vi "Tree Deep Copy Item.vi"(4 "Erase Target Tree":bool=TRUE, 6 "Parent Tag":string, 8 "error in":errorcluster, 9 "Target Tree Ref In":refnum<vi>, 10 "Target Item":string, 11 "Source Tree Ref In":refnum<vi>) -> (0 "error out":errorcluster, 1 "Target Tree Ref Out":refnum<vi>, 3 "Source Tree Ref Out":refnum<vi>)   [LabVIEW 2024]
uses:
  Tree Copy Single Item.vi
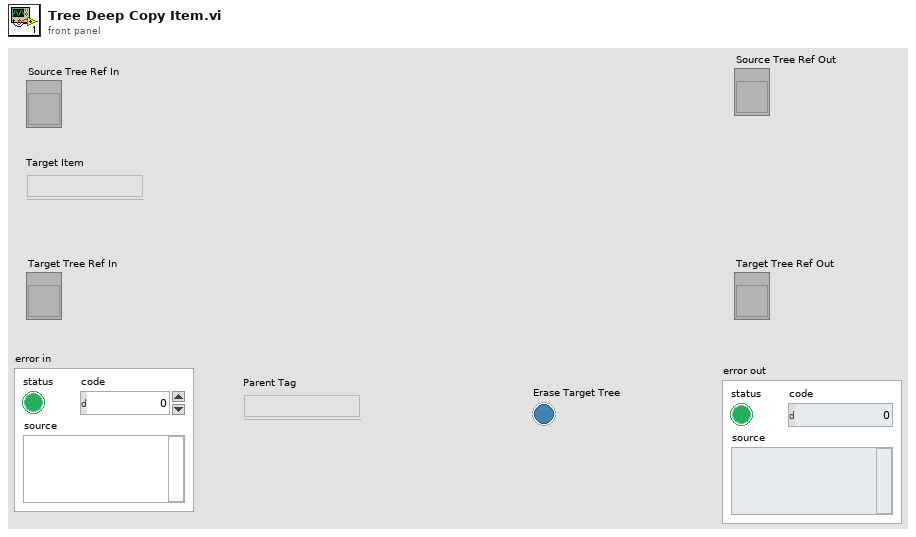
[diagram p1: front panel]
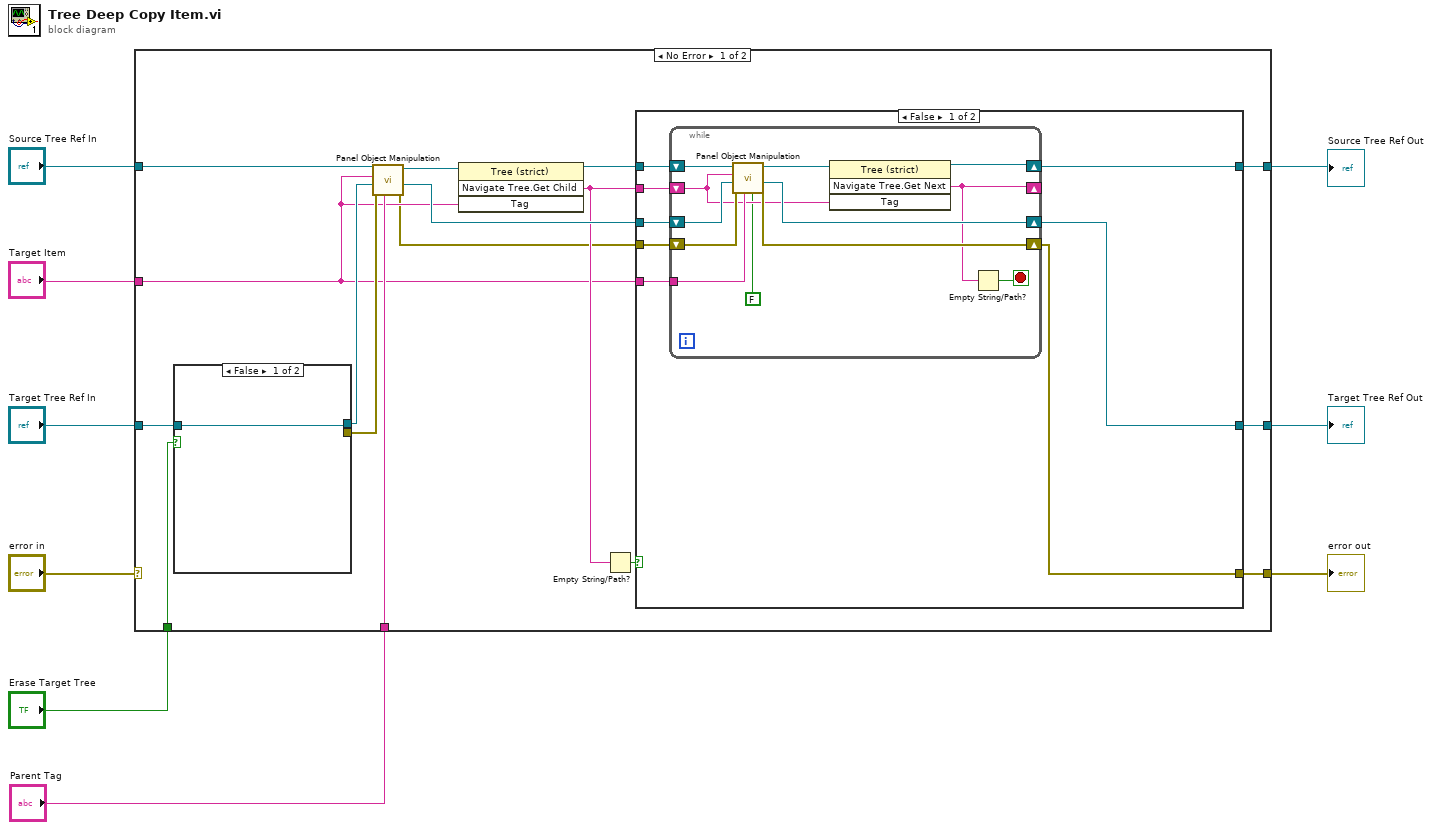
[diagram p0: block diagram]
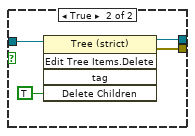
[diagram p3: hidden frame]
diagram:
  n1 = case shown="No Error" "error in" {
    selector: "error in" -> [_ w55]
    tunnel: [w10 w55] -> w8
    tunnel: "Target Tree Ref In" -> [w25 w53]
    tunnel: "Erase Target Tree" -> [w24 _]
    tunnel: "Target Item" -> [w12 _]
    tunnel: "Source Tree Ref In" -> [w23 w54]
    tunnel: "Parent Tag" -> [w20 _]
    tunnel: [w16 w54] -> w3
    tunnel: [w14 w53] -> w2
    frame No Error {
      n2 = case shown="False" w24 {
        tunnel: w25 -> [w48 w51]
        tunnel: [w48 w50] -> w22
        tunnel: [_ w49] -> w17
        frame False {
        }
        frame True {
          n3 = invoke class="Tree (strict)" method="Edit Tree Items.Delete"(reference=w51, "Delete Children"=TRUE ("Delete Children?")) -> (reference out=w50:refnum<vi>, error out=w49:errorcluster)  [unwired: 3 in, 3 out]
        }
      }
      n4 = call-poly "Panel Object Manipulation.vi"("Parent Tag"=w20, "error in"=w17, "Target Tree Ref In"=w22, "Target Item"=w12, "Source Tree Ref In"=w23) -> ("error out"=w11:errorcluster, "Target Tree Ref Out"=w15:refnum<vi>, "Source Tree Ref Out"=w21:refnum<vi>)  [unwired: 4 in]
      n5 = invoke class="Tree (strict)" method="Navigate Tree.Get Child"(reference=w21, "Tag"=w12) -> (reference out=w19:refnum<vi>, "Navigate Tree:Get Child"=w13:string)  [unwired: 2 in, 2 out]
      n6 = Empty String/Path?(string/path=w13) -> (empty?=w18:bool)
      n7 = case shown="False" w18 {
        tunnel: w19 -> [w33 w47]
        tunnel: [w29 w47] -> w16
        tunnel: w15 -> [w31 w46]
        tunnel: [w28 w46] -> w14
        tunnel: w13 -> [w32 _]
        tunnel: w12 -> [w30 _]
        tunnel: w11 -> [w27 _]
        tunnel: [w26 _] -> w10
        frame False {
          n8 = while {
            tunnel: w30 -> [w43]
            shift-right: [w38] -> w29
            shift-left: w33 -> [w45]
            shift-right: [w42] -> w28
            shift-left: w31 -> [w44]
            shift-right: [w40] -> w26
            shift-left: w27 -> [w41]
            shift-right: [w36] -> _
            shift-left: w32 -> [w37]
            stop <- w35 stop-if-true
            n9 = call-poly "Panel Object Manipulation.vi"("Erase Target Tree"=FALSE, "Parent Tag"=w43, "error in"=w41, "Target Tree Ref In"=w44, "Target Item"=w37, "Source Tree Ref In"=w45) -> ("error out"=w40:errorcluster, "Target Tree Ref Out"=w42:refnum<vi>, "Source Tree Ref Out"=w39:refnum<vi>)  [unwired: 3 in]
            n10 = invoke class="Tree (strict)" method="Navigate Tree.Get Next"(reference=w39, "Tag"=w37) -> (reference out=w38:refnum<vi>, "Navigate Tree:Get Next Item"=w36:string)  [unwired: 2 in, 2 out]
            n11 = Empty String/Path?(string/path=w36) -> (empty?=w35:bool)
          }
        }
        frame True {
        }
      }
    }
    frame Error {
    }
  }
  "Source Tree Ref Out" <- w3
  "Target Tree Ref Out" <- w2
  "error out" <- w8
